vi "Read Attributes.vi"(11 "Teller in":refnum<class "Teller.lvclass">) -> (2 "Attributes":refnum<class "Attributes.lvclass">)   [LabVIEW 2020, in "jettl.lvlib" / "Teller.lvclass"]
uses:
  Teller.lvclass
  Attributes/Attributes.lvclass
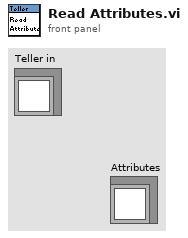
[diagram p1: front panel]
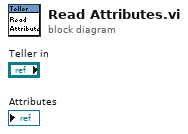
[diagram p0: block diagram]
diagram:
